vi "Get Testing Limits.vi"(0 "Program":string) -> (14 "Test Names":string[](array[string]), 15 "Low Limits":dbl[](array[numeric]), 16 "High Limits":dbl[](array[numeric]))   [LabVIEW 2023]
uses:
  <vilib>/Utility/file.llb/Read Delimited Spreadsheet (string).vi
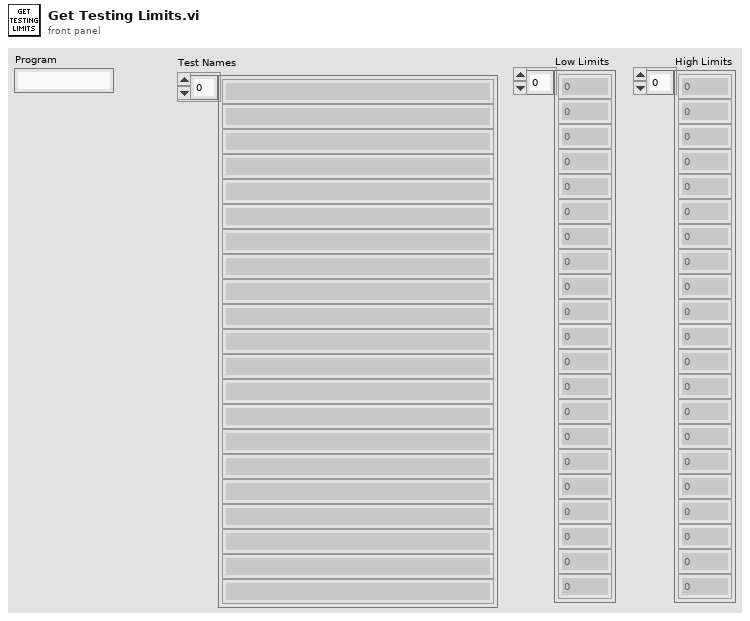
[diagram p1: front panel]
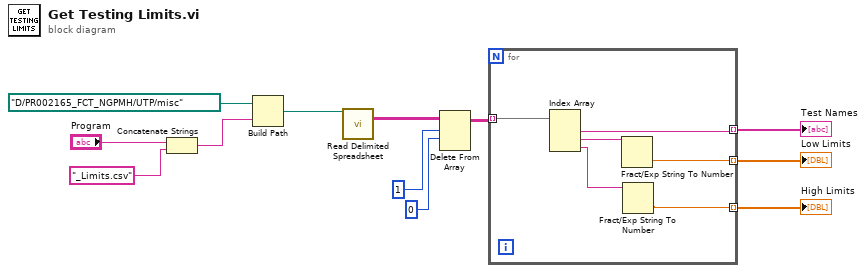
[diagram p0: block diagram]
diagram:
  n1 = Concatenate Strings("Program", "_Limits.csv" ("string")) -> (w6:string)
  n2 = Build Path(base path=path "D:/PR002165_FCT_NGPMH/UTP/misc" ("file path (dialog if empty)"), name or relative path=w6) -> (appended path=w11:path)
  n3 = call-poly <vilib>:"Read Delimited Spreadsheet.vi"("file path (dialog if empty)"=w11) -> ("all rows"=w4:string[][])  [unwired: 9 in, 5 out]
  n4 = Delete From Array(array=w4, length=1, index (row)=0) -> (array with subset deleted=w3:string[][])  [unwired: 1 in, 1 out]
  n5 = for {
    tunnel: w3 -> [w18] mode=indexing
    tunnel: [w15] -> w10 mode=indexing
    tunnel: [w14] -> w9 mode=indexing
    tunnel: [w13] -> w8 mode=indexing
    n6 = Index Array(array=w18) -> (element #1=w15:string, element #2=w17:string, element #3=w16:string)  [unwired: 3 in]
    n7 = Fract/Exp String To Number(string=w17) -> (number=w14:dbl)  [unwired: 3 in, 1 out]
    n8 = Fract/Exp String To Number(string=w16) -> (number=w13:dbl)  [unwired: 3 in, 1 out]
  }
  "Test Names" <- w10
  "Low Limits" <- w9
  "High Limits" <- w8
